vi "Pockels-Bundle modulation setup values.vi"(11 "Target time between ref triggers (ms)":dbl) -> (3 "Pockels modul. setup cluster":T1 {"Ref scan dwell time (us)" format="%#_13g"; "Pixels in ref image line" scale=2.0..80.0; "Dwell time (us)" format="%#_13g"; "Fill time (us)" format="%#_13g"; "Target time between ref triggers (ms)" min=0.5 max=10.0 step=0.5 format="%#_13g ms"; "Lines in ref image" scale=2.0..80.0; "Frame Size" items=["100X100"=100, "128X128"=128, "200X200"=200, "256X256"=256, "512X512"=512, "1024x1024"=1024, "2048x2048"=2048]})   [LabVIEW 2017]
uses:
  Typedefs/Pockels modulation setup cluster.ctl
  Typedefs/Frame Size.ctl
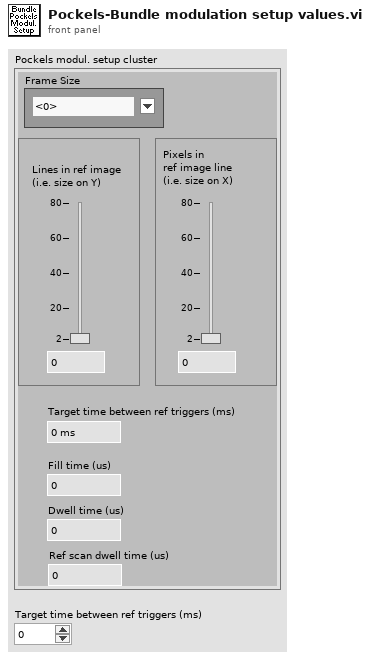
[diagram p1: front panel]
types:
  T1 = typedef "Pockels modulation setup cluster.ctl" = cluster{"Frame Size":T2, "Fill time (us)":dbl, "Dwell time (us)":dbl, "Ref scan dwell time (us)":dbl, "Lines in ref image":i16, "Pixels in ref image line":i16, "Target time between ref triggers (ms)":dbl}
  T2 = typedef "Frame Size.ctl" = u16
  T3 = typedef "AOL_Globals.ctl" = cluster{"Imaging Protocol":T4, "Number of POI":u16, "Number of Miniscans":u16, "Number of Trials":u16, "Number of Cycles ":u64, "# Averaged Frames":u16, "Laser power (%)":u8, "Pockels (V)":dbl, "Acquisition Length (sec)":dbl, "Fill time (us)":dbl, "POI Dwell time (us)":dbl, "Miniscan Dwell time per pixel (us)":dbl, "PMT 1":dbl, "PMT 2":dbl, "Back Apperture (mA)":dbl, "Frame Size":T2, "Center Frequency":dbl, "Field of View (norm)":dbl, "DwellTime (us)":dbl, "Wavelength (nm)":dbl, "Zoom":dbl, "AOL Z":dbl, "AOL Mode":T5, "GridXY":dbl, "GridZ":dbl, "TriggerPeriod (sec)":dbl, "Number of Pixels in Miniscan":u16, "Experiment folder path":path, "X centre":dbl, "Y centre":dbl, "Angle (degrees)":dbl, "Plane Mode":T6, "Threshold":u16[], "Regenerate Chirps":bool, "Rectangle ROI length (pixels)":u16, "Rectangle ROI height (pixels)":u16, "AOD fill":u16, "StartupDelay":i32, "Samples Wait after Trigger":u16, "Slip Cycle":u32, "Add Cycle":bool, "Functional Mode":T7, "Z Start":dbl, "Z Stop":dbl, "# Planes":i32}
  T4 = typedef "Imaging Protocols enum.ctl" = enum16{"AOL Z-Stack", "Motor Z Stack", "Functional Acquisition", "Single Plane Acquisition", "Volume Acquisition", "Live Imaging", "Live Plane Imaging", "Live Volume Imaging"}
  T5 = typedef "AOL modes.ctl" = enum16{"Raster", "Structural", "Pointing", "Mini Scan", "Alignment"}
  T6 = typedef "Plane Mode.ctl" = u16
  T7 = typedef "Functional Mode.ctl" = enum16{"Point", "Line", "Patch", "Plane", "Volume"}
  T8 = typedef "Ref DAQ Param.ctl" = cluster{"Full Frame Size":u16, "Ref Field of View":sgl, "Ref Zoom":i8, "Ref_dwellTime":sgl, "Ref X-pixels-per-line(Npxr)":i16, "Ref Y-lines-per-image(Npyr)":i16, "Ref Z-lines-per-image":i16, "Ref Scan Cycles":i32, "Ref threshold":u16, "Ref average":u16, "Sliding Average":bool, "proportioanl_scale":fxp<+,16,2>, "Integral_scale":fxp<+/-,16,12>, "proportioanl_scaleZ":fxp<+,16,2>, "Integral_scaleZ":fxp<+/-,16,12>, "Diff_threshold":fxp<+,16,2>, "Diff_threshold _z":fxp<+,16,2>, "scale":fxp<+,16,2>, "Control algorithm":T9, "New line trigger enabled":bool, "Slide Averaging":bool, "Ref count reset enabled":bool}
  T9 = typedef "Control algorithm.ctl" = enum16{"PID", "Kalman"}
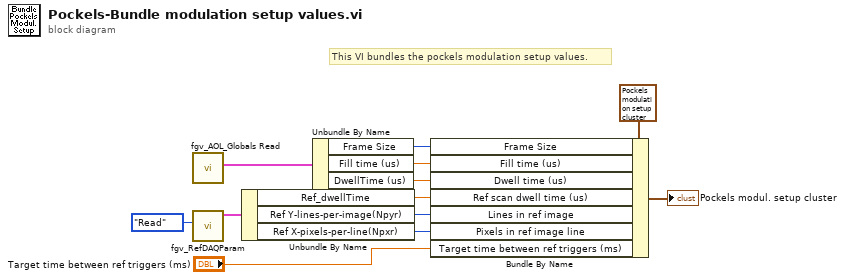
[diagram p0: block diagram]
diagram:
  # "This VI bundles the pockels modulation setup values."
  n1 = call "fgv_AOL_Globals Read.vi"() -> ("AOL_Globals"=w5:T3)  [unwired: 9 in, 2 out]
  n2 = call "fgv_RefDAQParam.vi"("Function"=enum16{"Initialize", "Write", "Read"}."Read" ("Status")) -> ("RefDAQParam"=w3:T8)  [unwired: 9 in, 1 out]
  n3 = Unbundle By Name(w3) -> ("Ref_dwellTime"=w10:sgl, "Ref Y-lines-per-image(Npyr)"=w11:i16, "Ref X-pixels-per-line(Npxr)"=w12:i16)
  n4 = Unbundle By Name(w5) -> ("Frame Size"=w6:T2, "Fill time (us)"=w8:dbl, "DwellTime (us)"=w9:dbl)
  n5 = Bundle By Name(cluster=T1 {"Frame Size"=512, "Fill time (us)"=16.0, "Dwell time (us)"=2.0, "Ref scan dwell time (us)"=25.399999618530273, "Lines in ref image"=0, "Pixels in ref image line"=16, "Target time between ref triggers (ms)"=0.1} ("Input values cluster"), "Frame Size"=w6, "Fill time (us)"=w8, "Dwell time (us)"=w9, "Ref scan dwell time (us)"=w10, "Lines in ref image"=w11, "Pixels in ref image line"=w12, "Target time between ref triggers (ms)"="Target time between ref triggers (ms)") -> (→"Pockels modul. setup cluster":T1)
